vi "triggered pulse and scope March 20 2017.vi"() -> ()   [LabVIEW 2014]
uses:
  <vilib>/Utility/file.llb/Write To Spreadsheet File (DBL).vi
  <instrlib>/Tektronix TDS 200 1000 2000 Series/Public/Configure/Configure Trigger (Edge).vi
  <instrlib>/Tektronix TDS 200 1000 2000 Series/Public/Data/Read (Multiple Waveforms).vi
  <vilib>/Waveform/WDTOps.llb/WDT Waveform to XY Pairs DBL.vi
  <instrlib>/Tektronix TDS 200 1000 2000 Series/Tektronix TDS 200 1000 2000 Series.lvlib
  <vilib>/Utility/file.llb/Write To Spreadsheet File (string).vi
panel:
  out "File path":path
  in  "Tektronix scope":T1={"Trigger"={" Source"=4, "Level (V)"=0.5, "Trigger Mode"=1, "Trigger Coupling"=1, "Trigger on?"=TRUE}, "Channel 1"={"V/div"=2.0, " offset (V)"=0.0}, "Channel 2"={"V/div"=2.0, " offset (V)"=0.0}, "Time base"={"s/div"=0.003, " offset (s)"=0.0}} {"Time base"."offset (s)" min=-1.0 max=1.0; "Time base"."s/div" min=2.5e-09 max=50.0; "Channel 2"."offset (V)" min=-20.0 max=20.0; "Channel 2"."V/div" min=0.02 max=50.0; "Channel 1"."offset (V)" min=-20.0 max=20.0; "Channel 1"."V/div" min=0.02 max=50.0; "Trigger"."Trigger Coupling" items=["AC", "DC", "HF Reject", "LF Reject", "Noise Reject"]; "Trigger"."Trigger Mode" items=["Auto", "Normal"]; "Trigger"."Level (V)" min=0.0 max=4.0; "Trigger"."Source" items=["Channel 1", "Channel 2", "Channel 3", "Channel 4", "External Input", "Attenuated External Input"]}
  out "Waveform Graph":waveform(dbl)[](graph)
  in  "Stop Button":bool
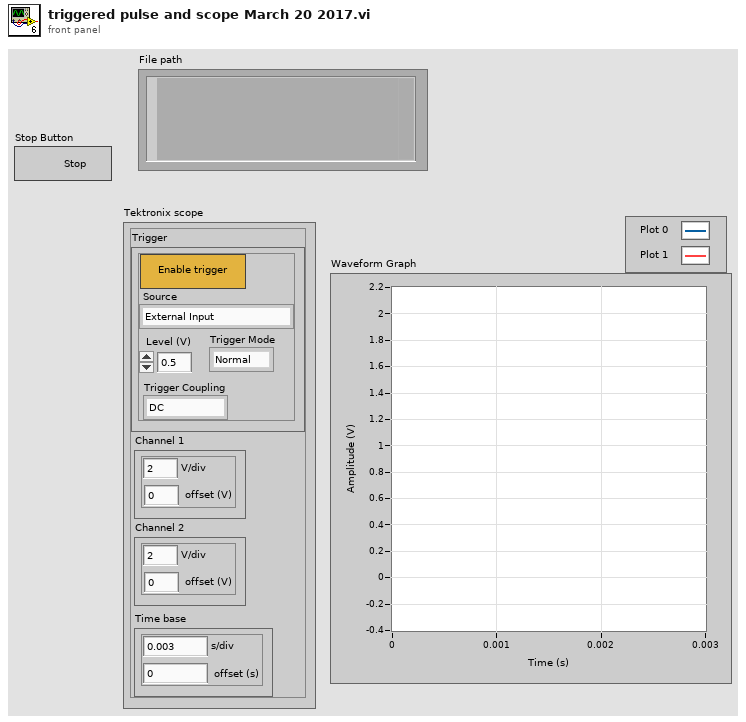
[diagram p1: front panel]
types:
  T1 = cluster{"Trigger":cluster{" Source":i32, "Level (V)":dbl, "Trigger Mode":i32, "Trigger Coupling":i32, "Trigger on?":bool}, "Channel 1":cluster{"V/div":dbl, " offset (V)":dbl}, "Channel 2":cluster{"V/div":dbl, " offset (V)":dbl}, "Time base":cluster{"s/div":dbl, " offset (s)":dbl}}
  T2 = cluster{" Source":i32, "Level (V)":dbl, "Trigger Mode":i32, "Trigger Coupling":i32, "Trigger on?":bool}
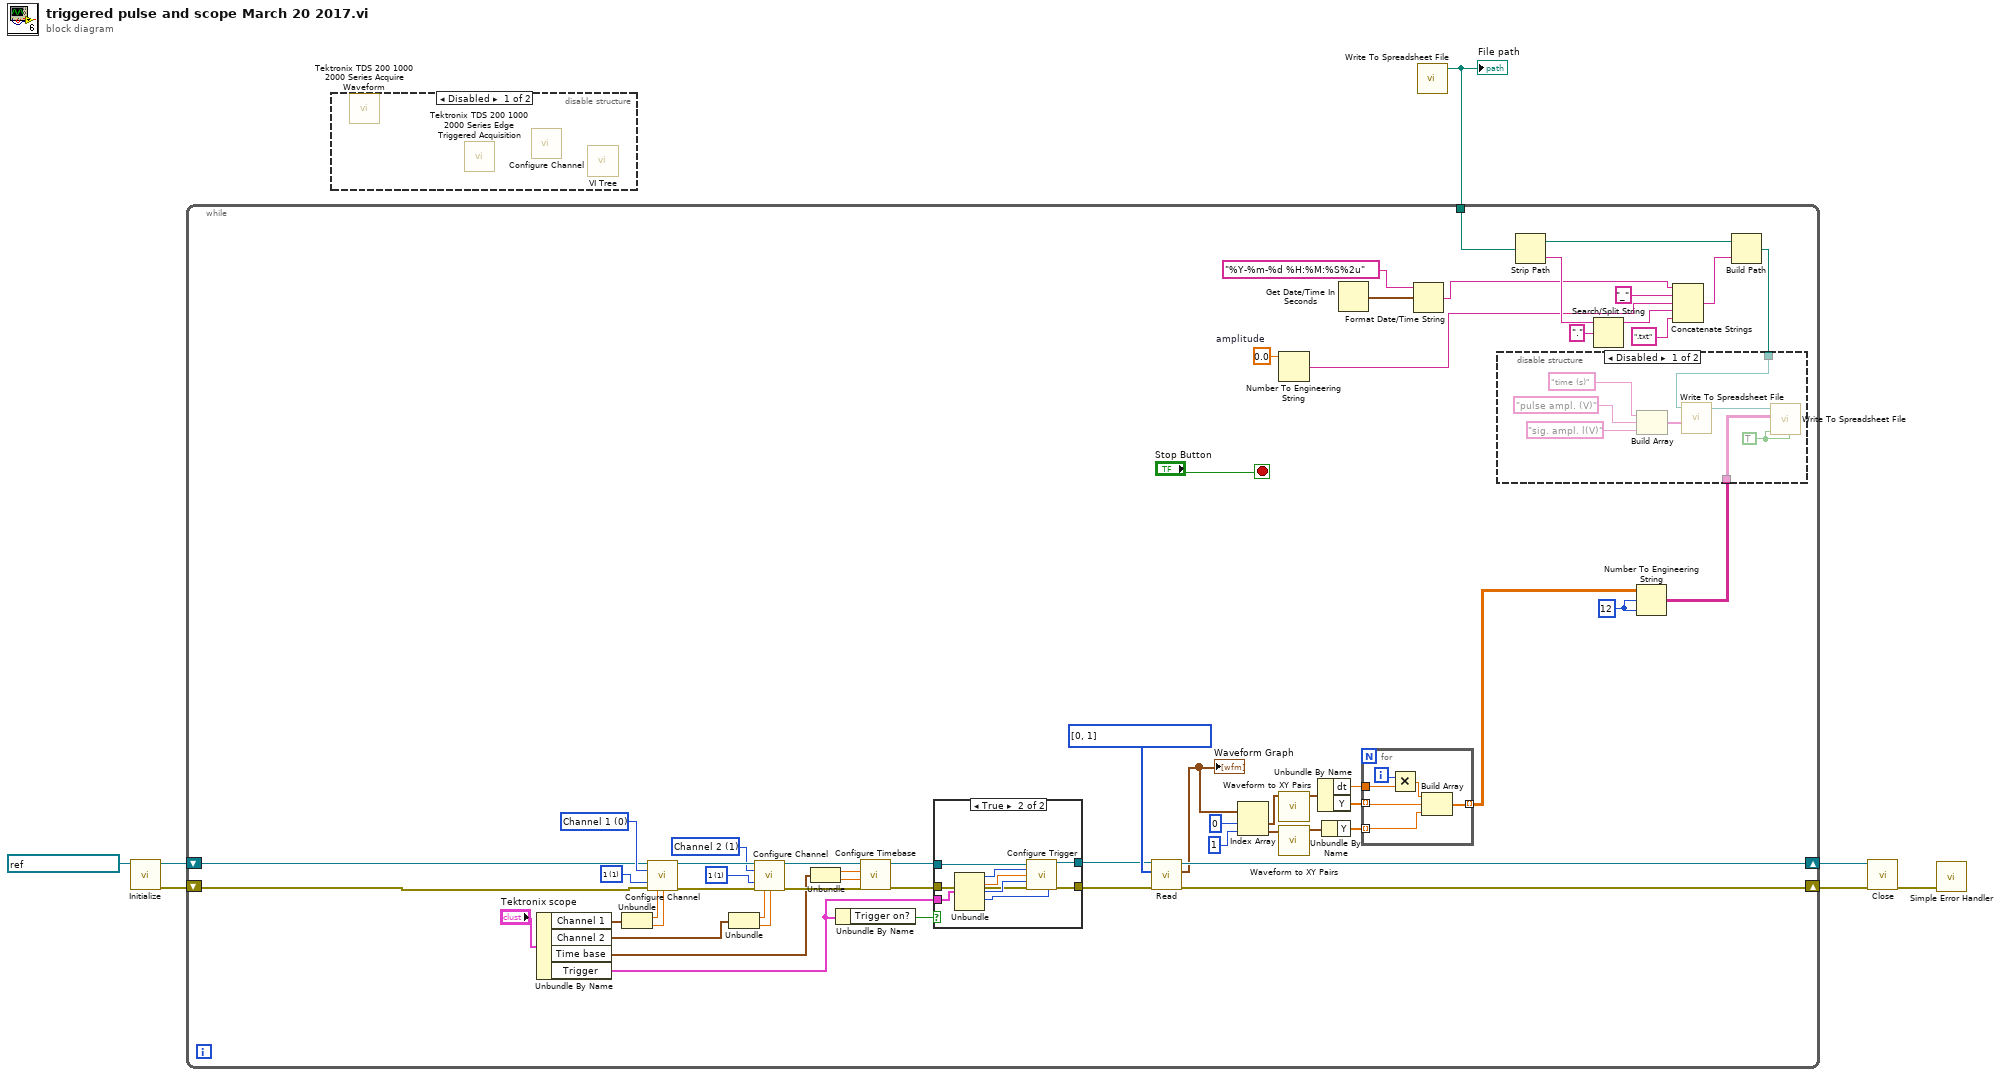
[diagram p0: block diagram]
diagram:
  n1 = call <instrlib>:"Initialize.vi"("VISA resource name"=refnum<visa-resource-name> "GPIB2::20::INSTR") -> ("error out"=w5:errorcluster, "VISA resource name out"=w6:refnum<visa-resource-name>)  [unwired: 9 in]
  n2 = disable-structure shown="Disabled" {
    frame Disabled {
      n3 = call "Tektronix TDS 200 1000 2000 Series Acquire Waveform.vi"() -> ()  [unwired: 1 in]
      n4 = call "Tektronix TDS 200 1000 2000 Series Edge Triggered Acquisition.vi"() -> ()  [unwired: 1 in]
      n5 = call <instrlib>:"Configure Channel.vi"() -> ()  [unwired: 14 in, 2 out]
      n6 = call "VI Tree.vi"() -> ()  [unwired: 12 in]
    }
    frame Enabled {
    }
  }
  n7 = call-poly <vilib>:"Write To Spreadsheet File.vi"() -> ("new file path (Not A Path if cancelled)"=w1:path)  [unwired: 8 in]
  "File path" <- w1
  n8 = while {
    shift-right: [w64] -> w7
    shift-left: w6 -> [w51]
    shift-right: [w63] -> w4
    shift-left: w5 -> [w9]
    tunnel: w1 -> [w18]
    stop <- "Stop Button" stop-if-true
    w10 = i16 12 ("width (-)")
    w13 = 0.0  # amplitude
    w41 = 1 items=["1"=1, "10"=10, "20"=20, "50"=50, "100"=100, "500"=500, "1000"=1000] ("Probe Attenuation (10: 10X)")
    w43 = 1 items=["1"=1, "10"=10, "20"=20, "50"=50, "100"=100, "500"=500, "1000"=1000] ("Probe Attenuation (10: 10X)")
    w42 = u16 1 items=["Channel 1", "Channel 2", "Channel 3", "Channel 4", "Math", "Reference A", "Reference B", "Reference C", "Reference D", "FFT"] ("Source (0: Channel 1)")
    w56 = u16 0 items=["Channel 1", "Channel 2", "Channel 3", "Channel 4", "Math", "Reference A", "Reference B", "Reference C", "Reference D", "FFT"] ("Source (0: Channel 1)")
    w62 = u16[] [0, 1] items=["Channel 1", "Channel 2", "Channel 3", "Channel 4", "Math", "Reference A", "Reference B", "Reference C", "Reference D", "FFT"] ("Channels")
    n9 = Unbundle By Name("Tektronix scope") -> ("Channel 1"=w38:cluster{"V/div":dbl, " offset (V)":dbl}, "Channel 2"=w37:cluster{"V/div":dbl, " offset (V)":dbl}, "Time base"=w36:cluster{"s/div":dbl, " offset (s)":dbl}, "Trigger"=w35:T2)
    n10 = Unbundle(w38) -> ("V/div"=w55:dbl, "offset (V)"=w54:dbl)
    n11 = call <instrlib>:"Configure Channel.vi"("VISA resource name"=w51, "Channel (0: Channel 1)"=w56, "Probe Attenuation (10: 10X)"=w43, "error in (no error)"=w9, "Vertical Range (10.0 V/div)"=w55, "Vertical Offset (0.0 divs)"=w54) -> ("VISA resource name out"=w61:refnum<visa-resource-name>, "error out"=w60:errorcluster)  [unwired: 8 in]
    n12 = Unbundle(w37) -> ("V/div"=w53:dbl, "offset (V)"=w52:dbl)
    n13 = call <instrlib>:"Configure Channel.vi"("VISA resource name"=w61, "Channel (0: Channel 1)"=w42, "Probe Attenuation (10: 10X)"=w41, "error in (no error)"=w60, "Vertical Range (10.0 V/div)"=w53, "Vertical Offset (0.0 divs)"=w52) -> ("VISA resource name out"=w50:refnum<visa-resource-name>, "error out"=w49:errorcluster)  [unwired: 8 in]
    n14 = Unbundle(w36) -> ("s/div"=w48:dbl, "offset (s)"=w47:dbl)
    n15 = Unbundle By Name(w35) -> ("Trigger on?"=w44:bool)
    n16 = call <instrlib>:"Configure Timebase.vi"("error in (no error)"=w49, "Position (0.0 s)"=w47, "Timebase (0.0005 s)"=w48, "VISA resource name"=w50) -> ("error out"=w45:errorcluster, "VISA resource name out"=w46:refnum<visa-resource-name>)  [unwired: 6 in]
    n17 = case shown="True" w44 {
      tunnel: w46 -> [w80 w85]
      tunnel: w45 -> [w79 w84]
      tunnel: [w80 w83] -> w29
      tunnel: [w79 w82] -> w28
      tunnel: w35 -> [_ w81]
      frame False {
      }
      frame True {
        n18 = Unbundle(w81) -> ("Source"=w86:i32, "Level (V)"=w87:dbl, "Trigger Mode"=w88:i32, "Trigger Coupling"=w89:i32)  [unwired: 1 out]
        n19 = call-poly <instrlib>:"Configure Trigger.vi"("VISA resource name"=w85, "Trigger Source (0: Channel 1)"=w86, "Trigger Level (0.0 V)"=w87, "Trigger Mode (0: Auto)"=w88, "error in (no error)"=w84, "Trigger Coupling (0: AC)"=w89) -> ("VISA resource name out"=w83:refnum<visa-resource-name>, "error out"=w82:errorcluster)  [unwired: 8 in]
      }
    }
    n20 = call-poly <instrlib>:"Read.vi"("error in (no error)"=w28, "Channels"=w62, "VISA resource name"=w29) -> ("error out"=w63:errorcluster, "Waveform Data"=w40:waveform(dbl)[], "VISA resource name out"=w64:refnum<visa-resource-name>)  [unwired: 6 in]
    "Waveform Graph" <- w40
    n21 = Index Array(array=w40, index #1=0 ("index"), index #2=1 ("index")) -> (element #1=w34:waveform(dbl), element #2=w57:waveform(dbl))
    n22 = Number To Engineering String(4:w13) -> (0:w14:string)  [unwired: 3 in]
    n23 = call-poly <vilib>:"Waveform to XY Pairs.vi"("waveform in"=w34) -> ("waveform out"=w33:waveform(dbl))  [unwired: 8 in, 2 out]
    n24 = call-poly <vilib>:"Waveform to XY Pairs.vi"("waveform in"=w57) -> ("waveform out"=w30:waveform(dbl))  [unwired: 8 in, 2 out]
    n25 = Unbundle By Name(w33) -> ("dt"=w32:dbl, "Y"=w31:dbl[])
    n26 = Unbundle By Name(w30) -> ("Y"=w26:dbl[])
    n27 = Get Date/Time In Seconds() -> (seconds since 1Jan1904=w27:timestamp)
    n28 = for {
      tunnel: w32 -> [w77]
      tunnel: w31 -> [w75] mode=indexing
      tunnel: [w74] -> w12 mode=indexing
      tunnel: w26 -> [w73] mode=indexing
      i -> [w78]
      n29 = Multiply(x=w78, y=w77) -> (x*y=w76:dbl)
      n30 = Build Array(w76, w75, w73) -> (w74:dbl[])
    }
    n31 = Format Date/Time String(time format string (%c)="%Y-%m-%d %H:%M:%S%2u", seconds (now)=w27) -> (date/time string=w16:string)  [unwired: 1 in]
    n32 = Strip Path(path=w18) -> (stripped path=w24:path, name=w23:string)
    n33 = Search/Split String(string=w23, search string/char (-)=".") -> (substring before match=w22:string)  [unwired: 1 in, 2 out]
    n34 = Number To Engineering String(2:w10, 3:w10, 4:w12) -> (0:w11:string[][])  [unwired: 1 in]
    n35 = Concatenate Strings(w16, "_" ("string"), w14, w22, ".txt" ("string")) -> (w20:string)
    n36 = Build Path(base path=w24, name or relative path=w20) -> (appended path=w25:path)
    n37 = disable-structure shown="Disabled" {
      disable-tunnel: w25 -> [w71 _]
      disable-tunnel: w11 -> [w65 _]
      frame Disabled {
        w67 = TRUE ("append to file? (new file:F)")
        n38 = Build Array("time (s)", "pulse ampl. (V)", "sig. ampl. l(V)") -> (w70:string[])
        n39 = call-poly <vilib>:"Write To Spreadsheet File.vi"("1D data"=w70, "file path (dialog if empty)"=w71) -> ("new file path (Not A Path if cancelled)"=w72:path)  [unwired: 6 in]
        n40 = call-poly <vilib>:"Write To Spreadsheet File.vi"("transpose? (no:F)"=w67, "append to file? (new file:F)"=w67, "2D data"=w65, "file path (dialog if empty)"=w72) -> ()  [unwired: 4 in, 1 out]
      }
      frame Enabled {
      }
    }
  }
  n41 = call <instrlib>:"Close.vi"("error in (no error)"=w4, "VISA resource name"=w7) -> ("error out"=w2:errorcluster)  [unwired: 9 in]
  n42 = call <vilib>:"Simple Error Handler.vi"("error in (no error)"=w2) -> ()  [unwired: 4 in, 5 out]
